vi "SVN Checkout Reload.vi"(8 "error in":errorcluster, 9 "ADT version":i32) -> (0 "error out":errorcluster, 1 "SVN Checkout output":string, 3 "Revision":i32, 4 "Success":bool, 6 "Successful Checkout":bool)   [LabVIEW 2011, in "Design Server.lvlib"]
uses:
  Design Server.lvlib
  Word cmd.ctl
  Mathcad15 cmds.ctl
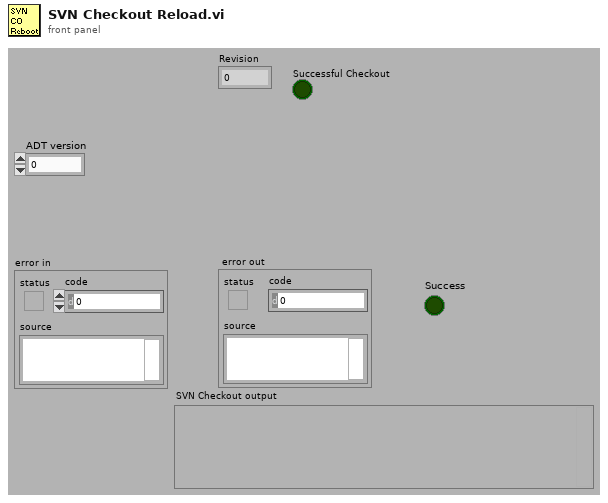
[diagram p1: front panel]
types:
  T1 = typedef "Design Server.lvlib/Mathcad15 cmds.ctl" = enum16{"Open Mathcad", "Execute Method", "Quit Mathcad"}
  T2 = typedef "Design Server.lvlib/Word cmd.ctl" = enum16{"Initialize", "Create Reports", "Quit"}
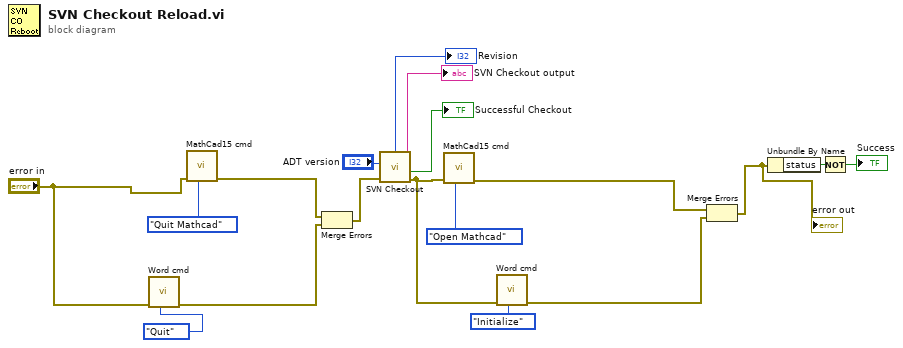
[diagram p0: block diagram]
diagram:
  n1 = call "Word cmd.vi"("Word cmd"=Word_cmd."Quit", "Error In (no error)"="error in") -> ("error out"=w9:errorcluster)  [unwired: 8 in, 1 out]
  n2 = call "MathCad15 cmd.vi"("Mathcad15 cmds"=Mathcad15_cmds."Quit Mathcad", "error in"="error in") -> ("first error out"=w8:errorcluster)  [unwired: 7 in, 2 out]
  n3 = Merge Errors(w8, w9) -> (w7:errorcluster)
  n4 = call "SVN Checkout.vi"("error in (no error)"=w7, "ADT version"="ADT version") -> ("error out"=w12:errorcluster, "Successful Checkout"=→"Successful Checkout":bool, "Revision"=→"Revision":i32, "standard output"=→"SVN Checkout output":string)  [unwired: 6 in]
  n5 = call "MathCad15 cmd.vi"("Mathcad15 cmds"=Mathcad15_cmds."Open Mathcad", "error in"=w12) -> ("first error out"=w2:errorcluster)  [unwired: 7 in, 2 out]
  n6 = call "Word cmd.vi"("Word cmd"=Word_cmd."Initialize", "Error In (no error)"=w12) -> ("error out"=w11:errorcluster)  [unwired: 8 in, 1 out]
  n7 = Merge Errors(w2, w11) -> (w10:errorcluster)
  "error out" <- w10
  n8 = Unbundle By Name(w10) -> ("status"=w15:bool)
  n9 = Not(x=w15) -> (.not. x?=→"Success":bool)
